vi "Sistema de ventilación-Para probar-Ramirez.vi"() -> ()   [LabVIEW 2023]
uses:
  <vilib>/MakerHub/LINX/Public/Peripherals/Analog/Analog Read 1 Chan.vi
  <vilib>/MakerHub/LINX/Public/Peripherals/Digital/Digital Write 1 Chan.vi
  <vilib>/MakerHub/LINX/Public/Peripherals/Analog/Analog Read N Chans.vi
  <vilib>/MakerHub/LINX/Public/Peripherals/Digital/Digital Write N Chans.vi
  <vilib>/MakerHub/LINX/Private/Local IO/LinxAnalogRead.vi
  <vilib>/MakerHub/LINX/Public/Utilities/Check Channel.vi
  <vilib>/MakerHub/LINX/Private/Local IO/LinxDigitalWrite.vi
  <vilib>/MakerHub/LINX/Public/Utilities/Open Serial.vi
  <vilib>/MakerHub/LINX/Public/Sensors/Motion/Servo/Servo Open One Channel.vi
  <vilib>/MakerHub/LINX/Public/Peripherals/Analog/Analog Write 1 Chan.vi
  <vilib>/MakerHub/LINX/Private/Utilties/Generate Error.vi
  <vilib>/MakerHub/LINX/Public/Sensors/Temperature/TMP3x/TMP35.vi
  <vilib>/MakerHub/LINX/Public/Sensors/Motion/Servo/Servo Set Pulse Width One Channel.vi
  <vilib>/MakerHub/LINX/Public/Sensors/Motion/Servo/Servo Close One Channel.vi
  <vilib>/MakerHub/LINX/LMH-LINX.lvlib
  <vilib>/MakerHub/LINX/Public/Sensors/Motion/Servo/Servo.lvlib
  <vilib>/MakerHub/LINX/Public/Sensors/Temperature/TMP3x/TMP3x.lvlib
panel:
  in  "Aire 2":dbl(knob) scale=-150.0..100.0
  in  "Aire":dbl(knob) scale=0.0..1000.0
  out "?":bool
  out "?":bool
  out "?":bool
  out "?":bool
  in  "?":bool
  out "Serevo Aire Angulo":string
  out "Serevo Temp Angulo":string
  in  "Serial Port":refnum<visa-resource-name>
  out "?":bool
  out "?":bool
  out "?":bool
  out "?":bool
  out "?":bool
  out "?":bool
  out "?":bool
  out "?":bool
  out "?":bool
  out "?":bool
  out "?":bool
  out "?":bool
  out "?":bool
  out "?":bool
  out "?":bool
  out "?":bool
  out "?":bool
  out "?":bool
  in  "?":bool
  out "Filtro de Calor":bool
  out "Filtro de Aire":bool
  out "Ppm del aire":dbl(knob) scale=0.0..1800.0
  out "Temperatura":dbl(slide) scale=0.0..60.0
  out "t [sec]":dbl
  out "Iteration No":i32
  in  "?":bool
  out "VI is running?":bool caption="ON/OFF"
  # "SISTEMA DE VENTILACIÓN DE DOBLE FLUJO"
  # "Temperatura"
  # "Entrada"
  # "Calidad del aire"
  # "Salida"
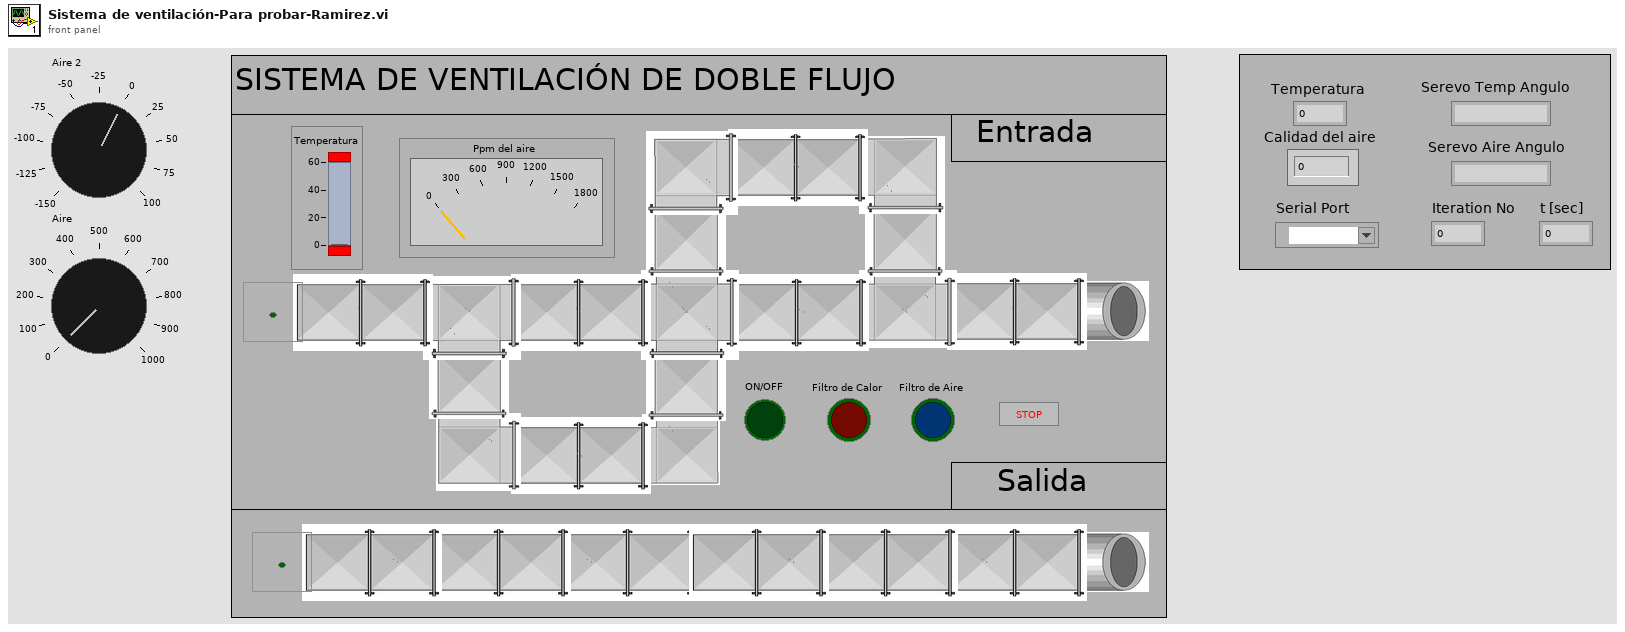
[diagram p1: front panel]
types:
  T1 = typedef "LMH-LINX.lvlib/LINX Ref.ctl" = cluster{"IO":T2, "Interface":T3, "LINX Device Config":T4}
  T2 = typedef "LMH-LINX.lvlib/Platform.ctl" = enum16{"Remote", "Local"}
  T3 = typedef "LMH-LINX.lvlib/Interface.ctl" = enum16{"Serial", "TCP"}
  T4 = typedef "LMH-LINX.lvlib/Device.lvlib/LINX Device Config.ctl" = cluster{"Interface":T3, "COM Port":refnum<visa-resource-name>, "TCP Configuration":T5, "Device Family":u8, "Device ID":u8, "Device Name":string, "TCP Ref":refnum<k5>, "Channels":T6}
  T5 = typedef "LMH-LINX.lvlib/Device.lvlib/TCP Config.ctl" = cluster{"IP Address":string, "Port":u16}
  T6 = typedef "LMH-LINX.lvlib/Channels.ctl" = cluster{"DI":u8[], "DO":u8[], "AI":u8[], "AO":u8[], "PWM":u8[], "QE":u8[], "UART":u8[], "I2C 2":u8[], "SPI":u8[], "CAN":u8[], "Servo":u8[], "AI Ref (V)":dbl, "AI Resolution (Bits)":u8, "AO Ref (V)":dbl, "AO Resolution (Bits)":u8}
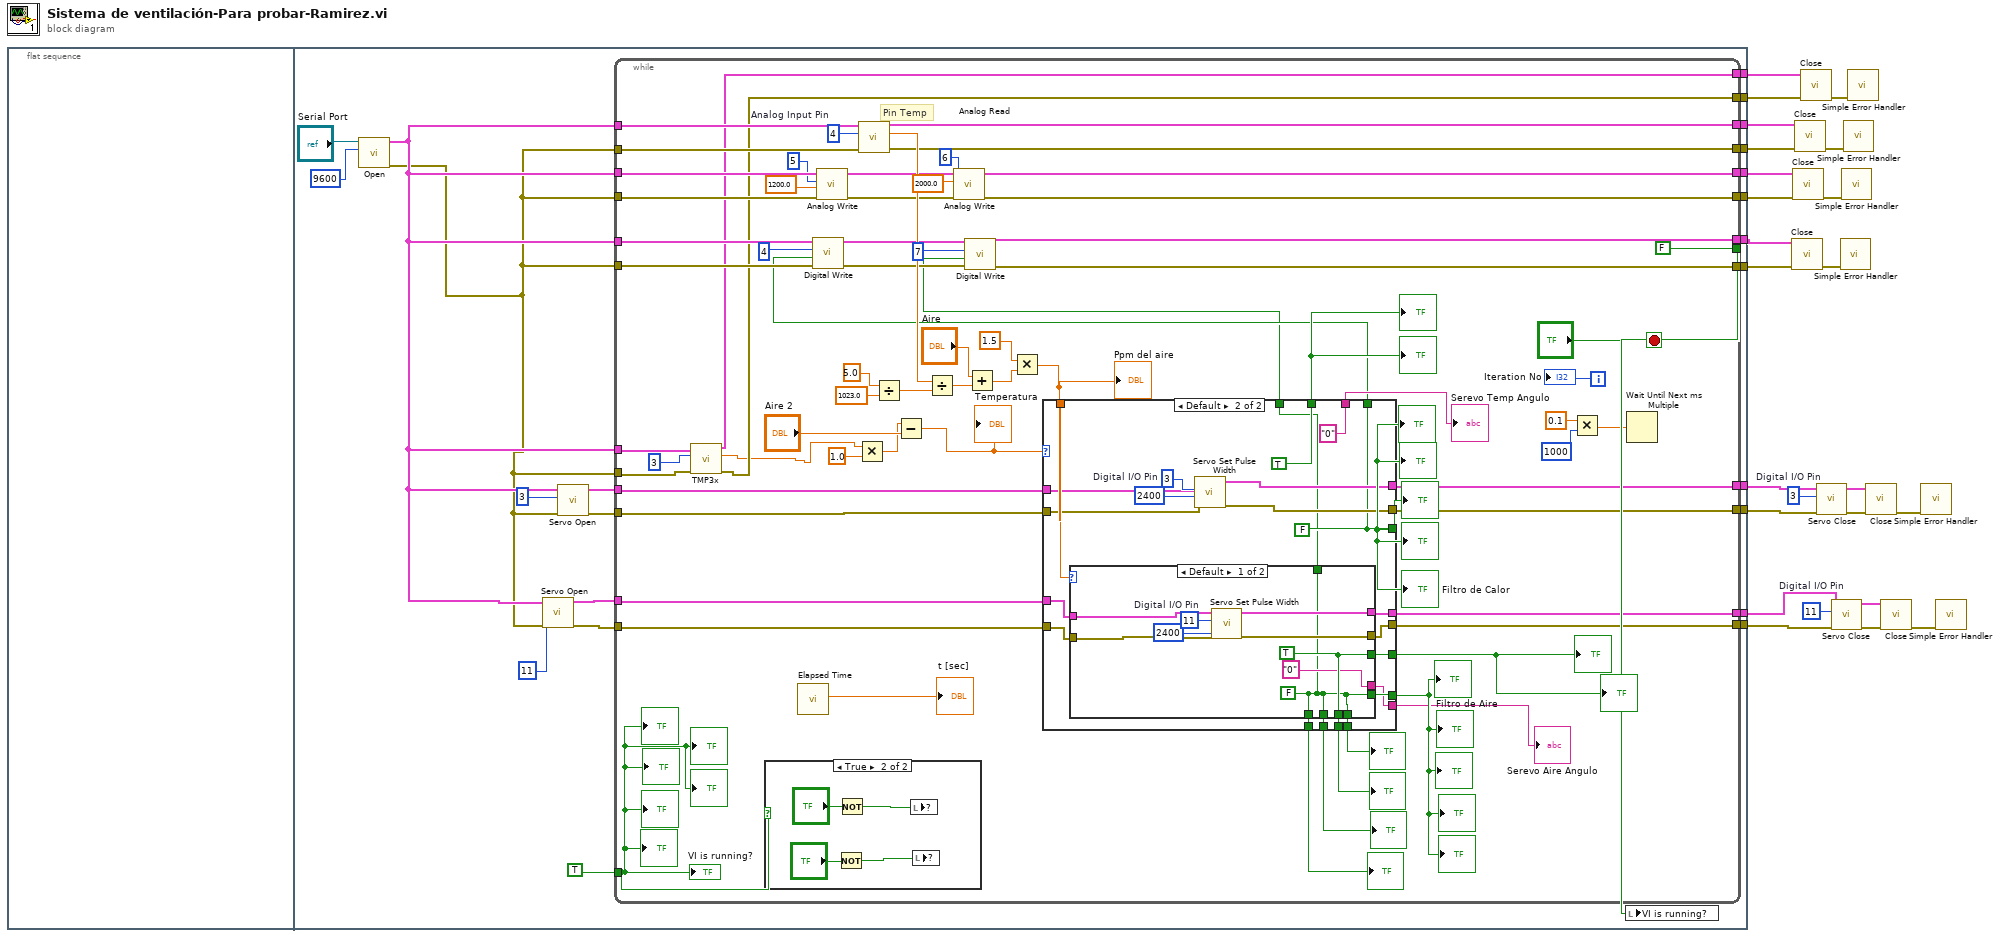
[diagram p0: block diagram]
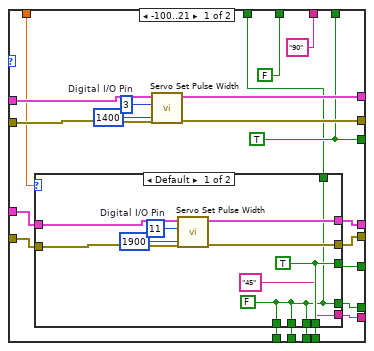
[diagram p2: hidden frame]
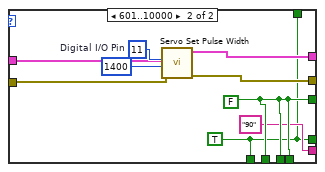
[diagram p3: hidden frame]
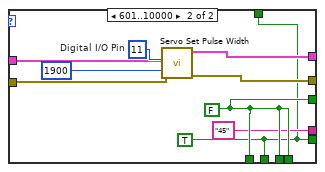
[diagram p4: hidden frame]
diagram:
  w7 = 11  # Digital I/O Pin
  w13 = 3  # Digital I/O Pin
  n1 = flat-sequence {
    tunnel: [w45] -> w24
    tunnel: [w43] -> w22
    tunnel: [w42] -> w20
    tunnel: [w41] -> w19
    tunnel: [w40] -> w17
    tunnel: [w39] -> w16
    tunnel: [w38] -> w1
    tunnel: [w37] -> w14
    tunnel: [w34] -> w9
    tunnel: [w33] -> w8
    tunnel: [w32] -> w3
    tunnel: [w31] -> w2
    frame #0 {
    }
    frame #1 {
      n2 = call-poly <vilib>:"Open.vi"("Baud Rate Override"=u32 9600, "Serial Port"="Serial Port") -> ("Error Out"=w27:errorcluster, "LINX Resource"=w29:T1)  [unwired: 7 in, 1 out]
      n3 = call-poly <vilib>:"Servo Open.vi"("Error In"=w27, "Servo Channel"=u8 11, "LINX Resource"=w29) -> ("Error Out"=w26:errorcluster, "LINX Resource"=w28:T1)  [unwired: 7 in]
      n4 = call-poly <vilib>:"Servo Open.vi"("Error In"=w27, "Servo Channel"=u8 3, "LINX Resource"=w29) -> ("Error Out"=w35:errorcluster, "LINX Resource"=w36:T1)  [unwired: 7 in]
      n5 = while {
        tunnel: [FALSE] -> w47
        tunnel: TRUE -> [w92]
        tunnel: w29 -> [w58]
        tunnel: [w59] -> w45
        tunnel: w27 -> [w61]
        tunnel: w29 -> [w111]
        tunnel: [w60] -> w43
        tunnel: w27 -> [w106]
        tunnel: [w104] -> w42
        tunnel: [w103] -> w41
        tunnel: w27 -> [w102]
        tunnel: w29 -> [w101]
        tunnel: [w94] -> w40
        tunnel: [w93] -> w39
        tunnel: w27 -> [w91]
        tunnel: w29 -> [w90]
        tunnel: [w85] -> w38
        tunnel: [w84] -> w37
        tunnel: w36 -> [w83]
        tunnel: w35 -> [w82]
        tunnel: [w81] -> w34
        tunnel: [w80] -> w33
        tunnel: w28 -> [w76]
        tunnel: w26 -> [w75]
        tunnel: [w74] -> w32
        tunnel: [w73] -> w31
        i -> [w113]
        stop <- "?" stop-if-true
        w105 = 4  # Analog Input Pin
        # "Pin Temp"
        n6 = call-poly <vilib>:"TMP3x.vi"("Error In"=w61, "Analog Channel"=u8 3, "LINX Resource"=w58) -> ("Error Out"=w60:errorcluster, "Temp C"=w52:dbl, "LINX Resource"=w59:T1)  [unwired: 6 in]
        n7 = case shown="True" w92 {
          frame False {
          }
          frame True {
            n8 = Not(x="?") -> (.not. x?=w199:bool)
            n9 = Not(x="?") -> (.not. x?=w201:bool)
            n10 = local write item#8(w201) -> ()
            n11 = local write item#30(w199) -> ()
          }
        }
        n12 = call "Elapsed Time"() -> ("Elapsed Time (s)"=→"t [sec]":dbl)  [unwired: 12 in, 7 out]
        n13 = call-poly <vilib>:"Analog Write.vi"("Error In"=w102, "AO Value"=1200.0, "AO Channel"=5, "LINX Resource"=w101) -> ("Error Out"=w95:errorcluster, "LINX Resource"=w96:T1)  [unwired: 6 in]
        n14 = Multiply(x=w52, y=1.0) -> (x*y=w50:dbl)
        n15 = call-poly <vilib>:"Analog Read.vi"("Error In"=w106, "Analog Channel"=w105, "LINX Resource"=w111) -> ("Error Out"=w103:errorcluster, "Voltage"=w108:dbl, "LINX Resource"=w104:T1)  [unwired: 5 in, 1 out]
        n16 = Divide(x=5.0, y=1023.0) -> (x/y=w107:dbl)
        n17 = Subtract(x=w50, y="Aire 2") -> (x-y=w49:dbl)
        "Temperatura" <- w49
        n18 = Divide(x=w108, y=w107) -> (x/y=w78:dbl)
        n19 = call-poly <vilib>:"Analog Write.vi"("Error In"=w95, "AO Value"=2000.0, "AO Channel"=6, "LINX Resource"=w96) -> ("Error Out"=w94:errorcluster, "LINX Resource"=w93:T1)  [unwired: 6 in]
        n20 = Add(x="Aire", y=w78) -> (x+y=w57:dbl)
        n21 = Multiply(x=1.5, y=w57) -> (x*y=w56:dbl)
        "Ppm del aire" <- w56
        n22 = case shown="Default" w49 {
          tunnel: w83 -> [w138 w178]
          tunnel: w82 -> [w137 w177]
          tunnel: [w136 w176] -> w81
          tunnel: [w135 w175] -> w80
          tunnel: [w120 w160] -> w77
          tunnel: [FALSE TRUE] -> w64
          tunnel: w76 -> [w130 w168]
          tunnel: w75 -> [w129 w167]
          tunnel: [w127 w169] -> w74
          tunnel: [w128 w170] -> w73
          tunnel: w56 -> [w131 w171]
          tunnel: [w133 w173] -> w72
          tunnel: [w132 w172] -> w71
          tunnel: [w126 w166] -> w70
          tunnel: [w123 w165] -> w69
          tunnel: [w124 w164] -> w68
          tunnel: [w125 w163] -> w67
          tunnel: ["90" ("Serevo Temp Angulo") "0" ("Serevo Temp Angulo")] -> w66
          tunnel: [w121 w161] -> w65
          tunnel: [w120 w160] -> w63
          tunnel: [w119 w159] -> w62
          frame -100..21 {
            w120 = TRUE
            w140 = 3  # Digital I/O Pin
            n23 = case shown="Default" w131 {
              tunnel: w130 -> [w147 w156]
              tunnel: w129 -> [w146 w155]
              tunnel: [w145 w154] -> w128
              tunnel: [w144 w153] -> w127
              tunnel: [w143 w152] -> w133
              tunnel: [w141 w150] -> w132
              tunnel: [w143 w152] -> w126
              tunnel: [w141 w150] -> w125
              tunnel: [w141 w152] -> w124
              tunnel: [w141 w152] -> w123
              tunnel: ["45" ("Serevo Aire Angulo") "90" ("Serevo Aire Angulo")] -> w121
              tunnel: [w141 w150] -> w119
              frame Default {
                w141 = FALSE
                w143 = TRUE
                w149 = 11  # Digital I/O Pin
                n24 = call-poly <vilib>:"Servo Set Pulse Width.vi"("Error In"=w146, "Pulse Width (uS)"=u16 1900, "Servo Channel"=w149, "LINX Resource"=w147) -> ("Error Out"=w144:errorcluster, "LINX Resource"=w145:T1)  [unwired: 6 in]
              }
              frame 601..10000 {
                w152 = FALSE
                w150 = TRUE
                w158 = 11  # Digital I/O Pin
                n25 = call-poly <vilib>:"Servo Set Pulse Width.vi"("Error In"=w155, "Pulse Width (uS)"=u16 1400, "Servo Channel"=w158, "LINX Resource"=w156) -> ("Error Out"=w153:errorcluster, "LINX Resource"=w154:T1)  [unwired: 6 in]
              }
            }
            n26 = call-poly <vilib>:"Servo Set Pulse Width.vi"("Error In"=w137, "Pulse Width (uS)"=u16 1400, "Servo Channel"=w140, "LINX Resource"=w138) -> ("Error Out"=w135:errorcluster, "LINX Resource"=w136:T1)  [unwired: 6 in]
          }
          frame Default {
            w160 = FALSE
            w180 = 3  # Digital I/O Pin
            n27 = case shown="Default" w171 {
              tunnel: w168 -> [w187 w197]
              tunnel: w167 -> [w186 w196]
              tunnel: [w185 w195] -> w170
              tunnel: [w184 w194] -> w169
              tunnel: [w183 w193] -> w173
              tunnel: [w181 w191] -> w172
              tunnel: [w181 w193] -> w166
              tunnel: [w183 w193] -> w165
              tunnel: [w181 w191] -> w164
              tunnel: [w181 w193] -> w163
              tunnel: ["0" ("Serevo Aire Angulo") "45" ("Serevo Aire Angulo")] -> w161
              tunnel: [w181 w191] -> w159
              frame Default {
                w181 = FALSE
                w183 = TRUE
                w189 = 11  # Digital I/O Pin
                n28 = call-poly <vilib>:"Servo Set Pulse Width.vi"("Error In"=w186, "Pulse Width (uS)"=u16 2400, "Servo Channel"=w189, "LINX Resource"=w187) -> ("Error Out"=w184:errorcluster, "LINX Resource"=w185:T1)  [unwired: 6 in]
              }
              frame 601..10000 {
                w193 = FALSE
                w191 = TRUE
                w198 = 11  # Digital I/O Pin
                n29 = call-poly <vilib>:"Servo Set Pulse Width.vi"("Error In"=w196, "Pulse Width (uS)"=u16 1900, "Servo Channel"=w198, "LINX Resource"=w197) -> ("Error Out"=w194:errorcluster, "LINX Resource"=w195:T1)  [unwired: 6 in]
              }
            }
            n30 = call-poly <vilib>:"Servo Set Pulse Width.vi"("Error In"=w177, "Pulse Width (uS)"=u16 2400, "Servo Channel"=w180, "LINX Resource"=w178) -> ("Error Out"=w175:errorcluster, "LINX Resource"=w176:T1)  [unwired: 6 in]
          }
        }
        "?" <- w68
        "?" <- w69
        "?" <- w67
        "?" <- w70
        "Serevo Temp Angulo" <- w66
        "Serevo Aire Angulo" <- w65
        "?" <- w77
        "?" <- w77
        "?" <- w77
        "?" <- w77
        "Filtro de Calor" <- w77
        "?" <- w64
        "?" <- w64
        "Filtro de Aire" <- w71
        "?" <- w71
        "?" <- w71
        "?" <- w71
        "?" <- w71
        "?" <- w72
        "?" <- w72
        n31 = call-poly <vilib>:"Digital Write.vi"("Error In"=w91, "Output Value"=w63, "DO Channel"=4, "LINX Resource"=w90) -> ("Error Out"=w86:errorcluster, "LINX Resource"=w87:T1)  [unwired: 6 in]
        n32 = call-poly <vilib>:"Digital Write.vi"("Error In"=w86, "Output Value"=w62, "DO Channel"=7, "LINX Resource"=w87) -> ("Error Out"=w84:errorcluster, "LINX Resource"=w85:T1)  [unwired: 6 in]
        n33 = Multiply(x=0.1, y=1000) -> (x*y=w116:dbl)
        n34 = Wait Until Next ms Multiple(millisecond multiple=w116) -> ()  [unwired: 1 out]
        "VI is running?" <- w92
        "Iteration No" <- w113
        "?" <- w92
        "?" <- w92
        "?" <- w92
        "?" <- w92
        "?" <- w92
        "?" <- w92
      }
      n35 = local write "VI is running?"(w47) -> ()
    }
  }
  n36 = call <vilib>:"Close.vi"("Error In"=w14, "LINX Resource"=w1) -> ("Error Out"=w15:errorcluster)  [unwired: 9 in]
  n37 = call <vilib>:"Close.vi"("Error In"=w17, "LINX Resource"=w16) -> ("Error Out"=w18:errorcluster)  [unwired: 9 in]
  n38 = call <vilib>:"Close.vi"("Error In"=w19, "LINX Resource"=w20) -> ("Error Out"=w21:errorcluster)  [unwired: 9 in]
  n39 = call <vilib>:"Close.vi"("Error In"=w22, "LINX Resource"=w24) -> ("Error Out"=w23:errorcluster)  [unwired: 9 in]
  n40 = call-poly <vilib>:"Servo Close.vi"("Error In"=w8, "Servo Channel"=w13, "LINX Resource"=w9) -> ("Error Out"=w11:errorcluster, "LINX Resource"=w12:T1)  [unwired: 7 in]
  n41 = call-poly <vilib>:"Servo Close.vi"("Error In"=w3, "Servo Channel"=w7, "LINX Resource"=w2) -> ("Error Out"=w5:errorcluster, "LINX Resource"=w6:T1)  [unwired: 7 in]
  n42 = call <vilib>:"Simple Error Handler.vi"("error in (no error)"=w15) -> ()  [unwired: 4 in, 5 out]
  n43 = call <vilib>:"Simple Error Handler.vi"("error in (no error)"=w18) -> ()  [unwired: 4 in, 5 out]
  n44 = call <vilib>:"Simple Error Handler.vi"("error in (no error)"=w21) -> ()  [unwired: 4 in, 5 out]
  n45 = call <vilib>:"Simple Error Handler.vi"("error in (no error)"=w23) -> ()  [unwired: 4 in, 5 out]
  n46 = call <vilib>:"Close.vi"("Error In"=w11, "LINX Resource"=w12) -> ("Error Out"=w10:errorcluster)  [unwired: 9 in]
  n47 = call <vilib>:"Close.vi"("Error In"=w5, "LINX Resource"=w6) -> ("Error Out"=w4:errorcluster)  [unwired: 9 in]
  n48 = call <vilib>:"Simple Error Handler.vi"("error in (no error)"=w10) -> ()  [unwired: 4 in, 5 out]
  n49 = call <vilib>:"Simple Error Handler.vi"("error in (no error)"=w4) -> ()  [unwired: 4 in, 5 out]
